vi "TriggerSnap.vi"(8 "error in (no error)":errorcluster, 9 "HardwareP":string[][](array[string]), 10 "Parameter":string[](array[string]), 11 "Refnum in":T2 caption="Session In") -> (0 "error out":errorcluster, 2 "ImageName":string[](array[string]), 3 "iMAGES":T1[](array[typedef]))   [LabVIEW 2015]
uses:
  <vilib>/userdefined/High Color/IMAQdx.ctl
  <vilib>/vision/Image Controls.llb/IMAQ Image.ctl
  <vilib>/vision/driver/IMAQdx.llb/IMAQdx Acquisition Mode.ctl
  <vilib>/vision/driver/IMAQdx.llb/IMAQdx Buffer Number Mode.ctl
  Global/PanelDisplayVI.vi
  Global/Global.vi
  <vilib>/vision/driver/NI_Vision_Acquisition_Software.lvlib
  <resource>/objmgr/imaqdx.rc
panel:
  in  "Boolean":bool
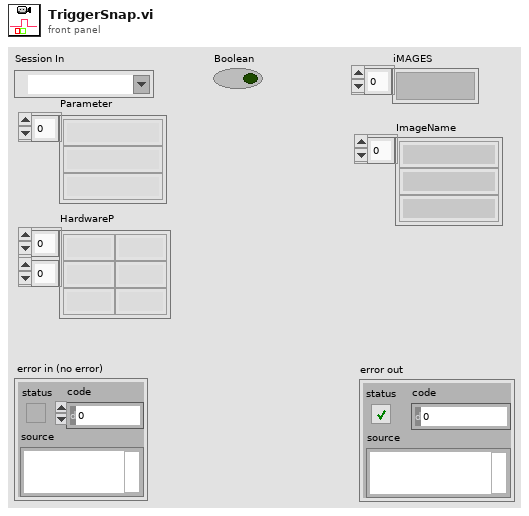
[diagram p1: front panel]
types:
  T1 = typedef "IMAQ Image.ctl" = refnum<image>
  T2 = typedef "IMAQdx.ctl" = refnum<k21>
  T3 = typedef "NI_Vision_Acquisition_Software.lvlib/IMAQdx Acquisition Mode.ctl" = enum32{"One Shot", "Continuous"}
  T4 = typedef "PanelDisplay.ctl" = cluster{"AlamStatus":refnum<vi>, "Reset&Clear":refnum<vi>, "AutoRun":refnum<vi>, "Pause/Continue":refnum<vi>, "USER":refnum<vi>, "Picture":refnum<vi>, "Home":refnum<vi>, "MachineParameter":refnum<vi>, "DataQuery":refnum<vi>, "UserLogin":refnum<vi>, "Stop":refnum<vi>, "AboutMachine":refnum<vi>, "menu reference":refnum<k9>, "RunningStatus_B":refnum<vi>, "CurrentProgram":refnum<vi>, "MeasurementData":refnum<vi>, "RunStatus":refnum<vi>, "SN":refnum<vi>, "OK/NG":refnum<vi>, "计数":refnum<vi>, "Image":refnum<vi>, "CT":refnum<vi>, "Slide":refnum<vi>, "Calculation":refnum<vi>, "PicCotrol":refnum<vi>, "ManualStart":refnum<vi>, "MeasurementDataNG":refnum<vi>, "Tab Control":refnum<vi>, "XY图":refnum<vi>, "波形图":refnum<vi>, "数据编号":refnum<vi>, "流线切换":refnum<vi>, "逆向电流":refnum<vi>}
  T5 = typedef "NI_Vision_Acquisition_Software.lvlib/IMAQdx Buffer Number Mode.ctl" = enum32{"Next", "Last", "Buffer Number", "Every", "Last New"}
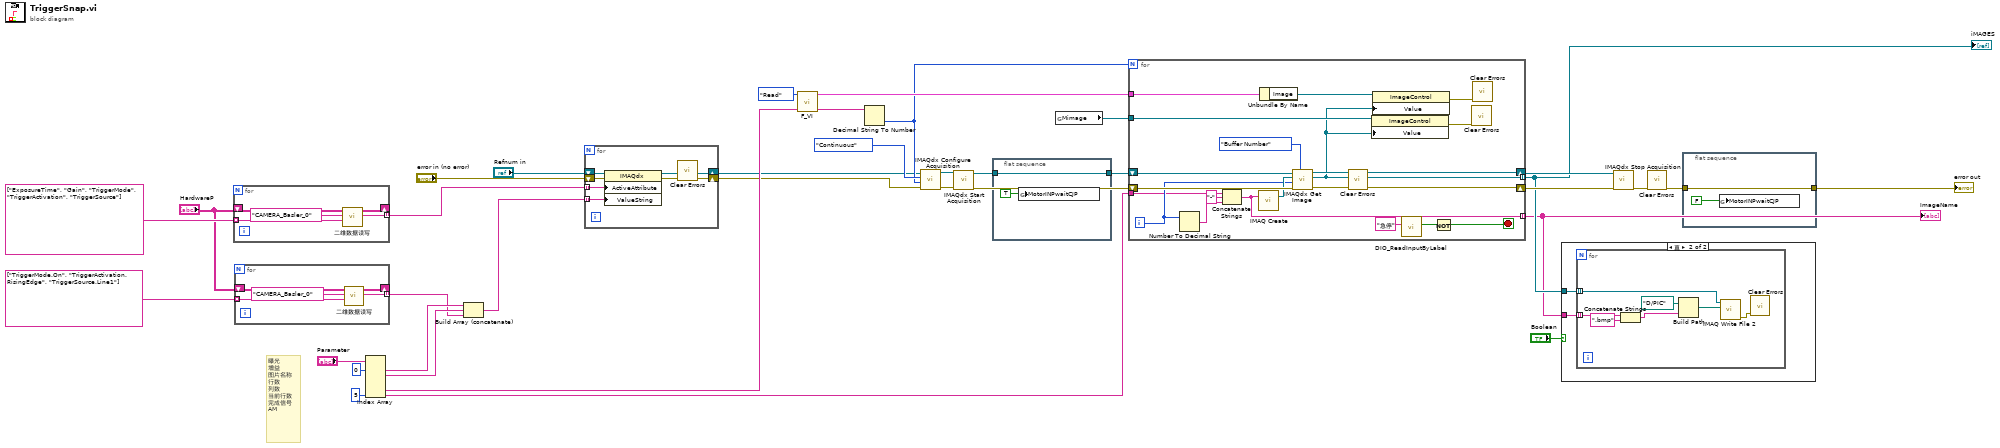
[diagram p0: block diagram]
diagram:
  # "曝光\n增益\n图片名称\n行数\n列数\n当前行数\n完成信号\nAM"
  n1 = for {
    tunnel: [w38] -> w3 mode=indexing
    tunnel: string[] ["ExposureTime", "Gain", "TriggerMode", "TriggerActivation", "TriggerSource"] -> [w37] mode=indexing
    shift-right: [w36] -> _
    shift-left: "HardwareP" -> [w40]
    n2 = call "二维数据读写.vi"("Name"=w37, "Item"="CAMERA_Basler_0", "ParameterDefine"=w40) -> ("Parameter Value"=w38:string, "ParameterDefineOUT"=w36:string[][])  [unwired: 5 in, 2 out]
  }
  n3 = for {
    tunnel: [w43] -> w2 mode=indexing
    tunnel: string[] ["TriggerMode.On", "TriggerActivation.RisingEdge", "TriggerSource.Line1"] -> [w42] mode=indexing
    shift-right: [w41] -> _
    shift-left: "HardwareP" -> [w45]
    n4 = call "二维数据读写.vi"("Name"=w42, "Item"="CAMERA_Basler_0", "ParameterDefine"=w45) -> ("Parameter Value"=w43:string, "ParameterDefineOUT"=w41:string[][])  [unwired: 5 in, 2 out]
  }
  n5 = Index Array(array="Parameter", index #1=0 ("index"), index #6=5 ("index")) -> (element #1=w9:string, element #2=w8:string, element #5=w32:string, element #6=w29:string)  [unwired: 4 in, 2 out]
  n6 = Build Array (concatenate)(w9, w8, w2) -> (w7:string[])
  n7 = for {
    tunnel: w3 -> [w52] mode=indexing
    tunnel: w7 -> [w49] mode=indexing
    shift-right: [w51] -> w12
    shift-left: "Refnum in" -> [w50]
    shift-right: [w47] -> w10
    shift-left: "error in (no error)" -> [w48]
    n8 = property class="IMAQdx"(reference=w50, error in=w48, "ActiveAttribute"=w52, "ValueString"=w49) -> (reference out=w51:T2, error out=w46:errorcluster)
    n9 = call <vilib>:"Clear Errors.vi"("error in (no error)"=w46) -> ("error out"=w47:errorcluster)  [unwired: 5 in, 1 out]
  }
  n10 = call-poly "F_VI.vi"("Step"=enum16{"Initial", "Read", "Write"}."Read") -> ("PanelDisplayOut"=w27:T4)  [unwired: 10 in]
  n11 = Decimal String To Number(string=w32) -> (number=w22:i32)  [unwired: 2 in, 1 out]
  n12 = call <vilib>:"IMAQdx Configure Acquisition.vi"("error in"=w10, "Number of Buffers"=w22, "Continuous?"=IMAQdx_Acquisition_Mode."Continuous", "Session In"=w12) -> ("error out"=w23:errorcluster, "Session Out"=w24:T2)  [unwired: 6 in]
  n13 = call <vilib>:"IMAQdx Start Acquisition.vi"("error in"=w23, "Session In"=w24) -> ("error out"=w26:errorcluster, "Session Out"=w15:T2)  [unwired: 8 in]
  n14 = flat-sequence {
    tunnel: w15 -> [w53]
    tunnel: [w53] -> w14
    frame #0 {
      n15 = global write "Global.vi" "MotorINPwaitCJP"(TRUE ("CJPwattingMotorINP")) -> ()
    }
  }
  n16 = global read "Global.vi" "Mimage"() -> (w1:refnum<vi>)
  n17 = for {
    N: w22 -> [_]
    shift-right: [w74] -> w35
    shift-left: w14 -> [w75]
    shift-right: [w65] -> w34
    shift-left: w26 -> [w73]
    tunnel: [w57] -> w21 mode=indexing
    tunnel: w29 -> [w67]
    tunnel: [w66] -> w20 mode=indexing
    tunnel: w27 -> [w62]
    tunnel: w1 -> [w58]
    i -> [w69]
    stop <- w59 stop-if-true
    n18 = Number To Decimal String(number=w69) -> (decimal integer string=w68:string)  [unwired: 1 in]
    n19 = Concatenate Strings(w67, "-" ("string"), w68) -> (w66:string)
    n20 = call "IMAQ Create"("Image Name"=w66) -> ("New Image"=w71:T1)  [unwired: 4 in, 1 out]
    n21 = Unbundle By Name(w62) -> ("Image"=w63:refnum<vi>)
    n22 = call <vilib>:"IMAQdx Get Image.vi"("Buffer Number Mode (Next)"=IMAQdx_Buffer_Number_Mode."Buffer Number", "error in"=w73, "Buffer Number In"=w69, "Image In"=w71, "Session In"=w75) -> ("error out"=w72:errorcluster, "Image Out"=w57:T1, "Session Out"=w74:T2)  [unwired: 3 in, 1 out]
    n23 = call <vilib>:"Clear Errors.vi"("error in (no error)"=w72) -> ("error out"=w65:errorcluster)  [unwired: 5 in, 1 out]
    n24 = property class="ImageControl"(reference=w58, "Value"=w57) -> (error out=w56:errorcluster)  [unwired: 1 in, 1 out]
    n25 = property class="ImageControl"(reference=w63, "Value"=w57) -> (error out=w55:errorcluster)  [unwired: 1 in, 1 out]
    n26 = call "DIO_ReadInputByLabel.vi"("Lable"="急停") -> ("Value"=w60:bool)  [unwired: 10 in]
    n27 = Not(x=w60) -> (.not. x?=w59:bool)
    n28 = call <vilib>:"Clear Errors.vi"("error in (no error)"=w56) -> ()  [unwired: 5 in, 2 out]
    n29 = call <vilib>:"Clear Errors.vi"("error in (no error)"=w55) -> ()  [unwired: 5 in, 2 out]
  }
  "iMAGES" <- w21
  "ImageName" <- w20
  n30 = case shown="真" "Boolean" {
    tunnel: w21 -> [_ w77]
    tunnel: w20 -> [_ w76]
    frame False {
    }
    frame True {
      n31 = for {
        tunnel: w77 -> [w80] mode=indexing
        tunnel: w76 -> [w83] mode=indexing
        n32 = Concatenate Strings(w83, ".bmp" ("string")) -> (w81:string)
        n33 = Build Path(base path=path "D:/PIC", name or relative path=w81) -> (appended path=w79:path)
        n34 = call-poly "IMAQ Write File 2"("File Path"=w79, "Image"=w80) -> ("error out"=w78:errorcluster)  [unwired: 8 in, 1 out]
        n35 = call <vilib>:"Clear Errors.vi"("error in (no error)"=w78) -> ()  [unwired: 5 in, 2 out]
      }
    }
  }
  n36 = call <vilib>:"IMAQdx Stop Acquisition.vi"("error in"=w34, "Session In"=w35) -> ("error out"=w18:errorcluster)  [unwired: 8 in, 1 out]
  n37 = call <vilib>:"Clear Errors.vi"("error in (no error)"=w18) -> ("error out"=w17:errorcluster)  [unwired: 5 in, 1 out]
  n38 = flat-sequence {
    tunnel: w17 -> [w86]
    tunnel: [w86] -> w16
    frame #0 {
      n39 = global write "Global.vi" "MotorINPwaitCJP"(FALSE ("CJPwattingMotorINP")) -> ()
    }
  }
  "error out" <- w16
